vi "Parse-attribute.vi"(8 "error in (no error)":errorcluster, 10 "String in":string, 11 "Time in":refnum<class "Time.lvclass">) -> (0 "error out":errorcluster, 1 "Valid attribute?":bool, 2 "Remaining string":string, 3 "Time out":refnum<class "Time.lvclass">)   [LabVIEW 2013, in "HardwareCharacterization.lvlib" / "Time.lvclass"]
uses:
  Time.lvclass
  Time.lvclass/Time.ctl
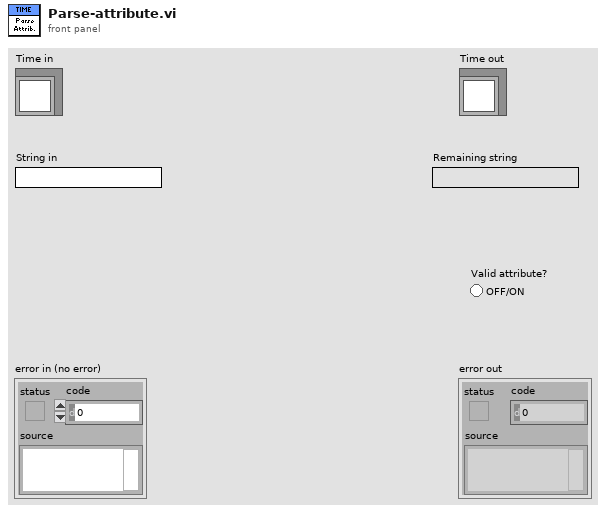
[diagram p1: front panel]
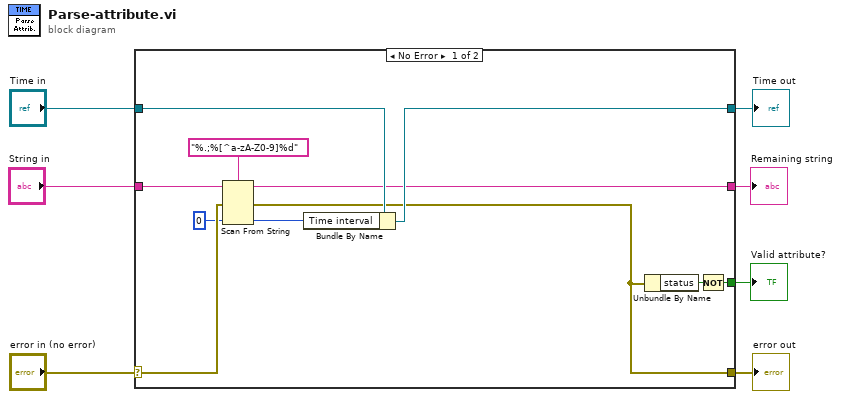
[diagram p0: block diagram]
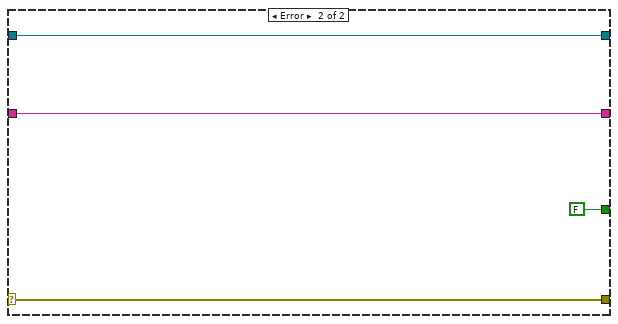
[diagram p2: hidden frame]
diagram:
  n1 = case shown="No Error" "error in (no error)" {
    selector: "error in (no error)" -> [w14 w22]
    tunnel: [w9 w22] -> w6
    tunnel: [w11 w21] -> w4
    tunnel: "Time in" -> [w12 w21]
    tunnel: "String in" -> [w15 w19]
    tunnel: [w10 w19] -> w2
    tunnel: [w8 FALSE] -> w1
    frame No Error {
      n2 = Scan From String(format string="%.;%[^a-zA-Z0-9]%d", input string=w15, error in=w14, default 2=i64 0 ("default value 2")) -> (remaining string=w10:string, error out=w9:errorcluster, output 2=w16:i64)  [unwired: 3 in, 1 out]
      n3 = Bundle By Name(cluster=w12, "Time interval"=w16) -> (w11:refnum<class "Time.lvclass">)
      n4 = Unbundle By Name(w9) -> ("status"=w17:bool)
      n5 = Not(x=w17) -> (.not. x?=w8:bool)
    }
    frame Error {
    }
  }
  "error out" <- w6
  "Time out" <- w4
  "Remaining string" <- w2
  "Valid attribute?" <- w1
